vi "Closed Hood Control.vi"(2 "Time Delay":dbl) -> ()   [LabVIEW 2011]
uses:
  System Set Points and States.vi
  <vilib>/addons/control/pid/pid.llb/PID (DBL).vi
  <vilib>/addons/control/pid/NI_PID_pid.lvlib
panel:
  out "Target Voltage":dbl
  in  "D":dbl
  in  "I":dbl
  in  "P":dbl=0.05 step=0.001
  out "Error":dbl
  out "Pot Voltage":dbl
  # "Tuning Controls"
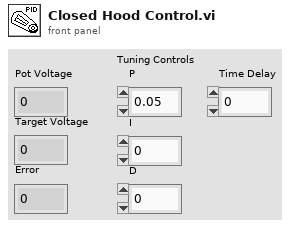
[diagram p1: front panel]
types:
  T1 = typedef "WPI_AnalogChannelDevRef.ctl" = cluster{"DevStatus":errorcluster, "Analog Module":T2, "Analog Channel":T3}
  T2 = typedef "FPGA_TypedefAnalogModule.ctl" = enum16{"Analog Module 1", "Analog Module 2"}
  T3 = typedef "FPGA_AIChannel.ctl" = enum8{"AI 1", "AI 2", "AI 3", "AI 4", "AI 5", "AI 6", "AI 7", "AI 8", "Invalid"}
  T4 = typedef "WPI_MotorControlDeviceRef.ctl" = cluster{"DeviceStatus":errorcluster, "Type":enum16{"PWM", "CAN"}, "PWM":cluster{"Digital Module":T5, "PWM Channel":T6, "DeadBand":T7}, "CAN":cluster{"Device Number":u8, "Control Mode":T8, "Semaphore":T9, "Max Vout":dbl}, "Invert":bool, "TransformRef":T10, "InvTransformRef":T10}
  T5 = typedef "FPGA_TypedefDigitalModule.ctl" = enum16{"Digital Module 1", "Digital Module 2"}
  T6 = typedef "FPGA_DIOPWMChannel.ctl" = enum8{"PWM 1", "PWM 2", "PWM 3", "PWM 4", "PWM 5", "PWM 6", "PWM 7", "PWM 8", "PWM 9", "PWM 10", "Invalid"}
  T7 = typedef "WPI_PWMDeadband.ctl" = cluster{"Name":string, "maxPositivePwm":i32, "minPositivePwm":i32, "centerPwm":i32, "maxNegativePwm":i32, "minNegativePwm":i32, "angularRange":u16}
  T8 = typedef "WPI_CANJaguar_ControlMode.ctl" = enum8{"Percent VBus", "Current", "Speed", "Position", "Voltage"}
  T9 = typedef "Semaphore RefNum" = refnum<k1>
  T10 = typedef "WPI_PWMTransform_ConPane.ctl" = refnum<vi>
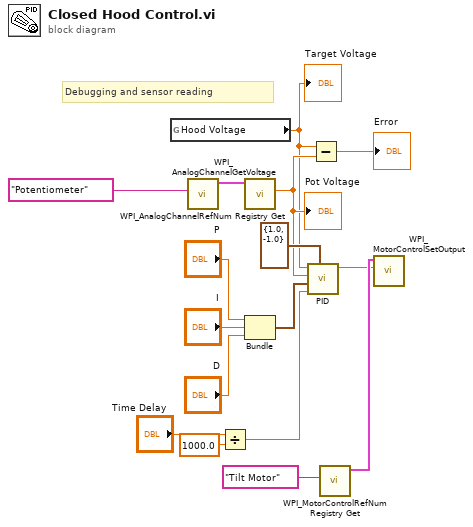
[diagram p0: block diagram]
diagram:
  # "Debugging and sensor reading"
  n1 = global read "System Set Points and States.vi" "Hood Voltage"() -> (w7:dbl)
  "Target Voltage" <- w7
  n2 = call <vilib>:"WPI_AnalogChannelRefNum Registry Get.vi"("refnum name"="Potentiometer") -> ("AIDeviceRef"=w14:T1)  [unwired: 9 in, 1 out]
  n3 = Divide(x="Time Delay", y=1000.0) -> (x/y=w1:dbl)
  n4 = call <vilib>:"WPI_AnalogChannelGetVoltage.vi"("AIDeviceRef"=w14) -> ("Voltage"=w13:dbl)  [unwired: 8 in, 2 out]
  "Pot Voltage" <- w13
  n5 = Bundle("P"="P", "I"="I", "D"="D") -> (w8:cluster{"P":dbl, "I":dbl, "D":dbl})  [unwired: 1 in]
  n6 = call-poly <vilib>:"PID.vi"("output range"=cluster{"output high":dbl, "output low":dbl} {"output high"=1.0, "output low"=-1.0}, "dt (s)"=w1, "PID gains"=w8, "process variable"=w13, "setpoint"=w7) -> ("output"=w4:dbl)  [unwired: 5 in, 1 out]
  n7 = Subtract(x=w7, y=w13) -> (x-y=→"Error":dbl)
  n8 = call <vilib>:"WPI_MotorControlRefNum Registry Get.vi"("refnum name"="Tilt Motor") -> ("MotorControlDevRef"=w5:T4)  [unwired: 9 in, 1 out]
  n9 = call <vilib>:"WPI_MotorControlSetOutput.vi"("Output"=w4, "MotorControlDevRef"=w5) -> ()  [unwired: 8 in, 2 out]
